vi "文件读取测试.vi"() -> ()   [LabVIEW 2012]
panel:
  in  "数值":i32
  out "输出 4":dbl
  out "输出 2":dbl
  in  "文件路径（使用对话框）":path
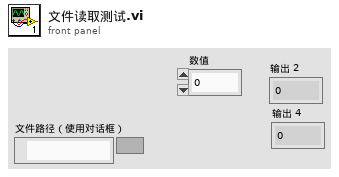
[diagram p1: front panel]
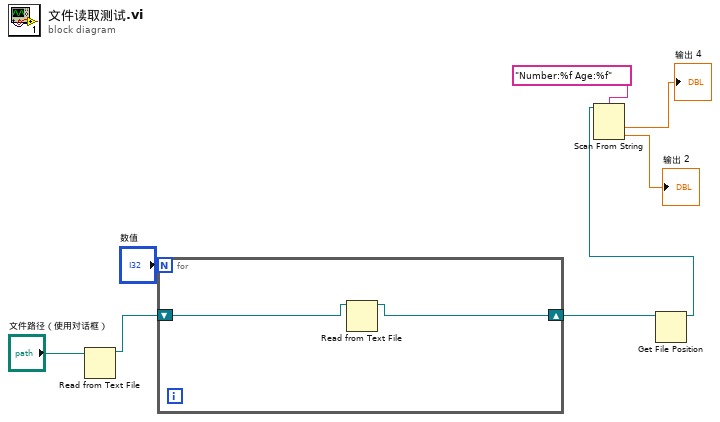
[diagram p0: block diagram]
diagram:
  n1 = Read from Text File(file (use dialog)="文件路径（使用对话框）") -> (refnum out=w3:refnum<file>)  [unwired: 3 in, 3 out]
  n2 = for {
    N: "数值" -> [_]
    shift-right: [w9] -> w2
    shift-left: w3 -> [w10]
    n3 = Read from Text File(file (use dialog)=w10) -> (refnum out=w9:refnum<file>)  [unwired: 3 in, 3 out]
  }
  n4 = Get File Position(7:w2) -> (3:w1:refnum<file>)  [unwired: 1 in, 2 out]
  n5 = Scan From String("Number:%f Age:%f" ("格式字符串"), w1) -> (output 1=→"输出 4":dbl, output 2=→"输出 2":dbl)  [unwired: 3 in, 2 out]
